vi "brc_daq_connect_module.vi"(8 "error in (no error)":errorcluster, 11 "index":i32) -> (0 "error out":errorcluster, 3 "return_value":i32)   [LabVIEW 2019, in "BRC-DAQ.lvlib"]
uses:
  BRC-DAQ.lvlib
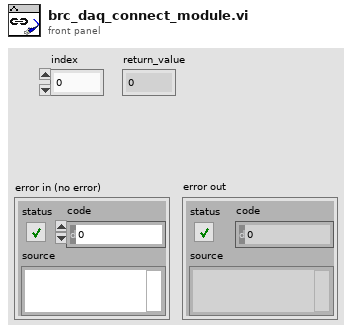
[diagram p1: front panel]
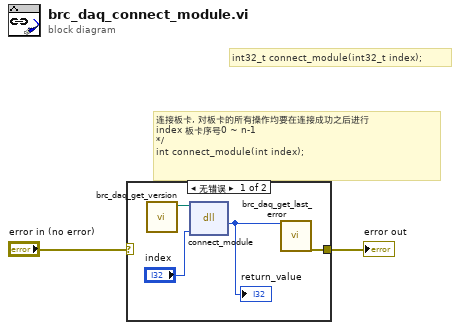
[diagram p0: block diagram]
diagram:
  # "int32_t connect_module(int32_t index);"
  # "连接板卡, 对板卡的所有操作均要在连接成功之后进行\nindex 板卡序号0 ~ n-1\n*/\nint connect_module(int index);"
  n1 = case shown="无错误" "error in (no error)" {
    selector: "error in (no error)" -> [_ w7]
    tunnel: [w4 w7] -> w2
    frame No Error {
      n2 = call "brc_daq_get_version.vi"() -> ("dll path"=w3:path)  [unwired: 11 in]
      n3 = dll-call lib="E:/01 BRC project/04BRC-daq/04 Drive/DAQ-x64/DLL/brc_daq_sdk.dll" fn="connect_module"(path in=w3, "index"="index") -> ("return type"=w5:i32)  [unwired: 3 in, 2 out]
      "return_value" <- w5
      n4 = call "brc_daq_get_last_error.vi"("return_value"=w5) -> ("error out"=w4:errorcluster)  [unwired: 18 in]
    }
    frame Error {
    }
  }
  "error out" <- w2
